vi "Drawing Proof Of Concept Early.vi"() -> ()   [LabVIEW 2021]
uses:
  <vilib>/Utility/inputDevices.llb/mouseAcquire.vi
  <vilib>/Utility/inputDevices.llb/closeMouse.vi
panel:
  in  "Clear Drawing":bool
  out "Robot Drawn So Far":cluster{i32[], i32[]}[](graph)
  in  "Cancel Drawing Queue":bool
  out "Obstacle Detected":bool
  out "Robot Vertical":dbl
  out "Robot Horizontal":dbl
  out "Chalk Force Readout":dbl
  out "Current Mouse Coordinates":T1
  out "Drawing":cluster{i32[], i32[]}[](graph)
  out "Mouse Status":cluster{"Clicked?":bool}
  in  "Emergency Stop":bool
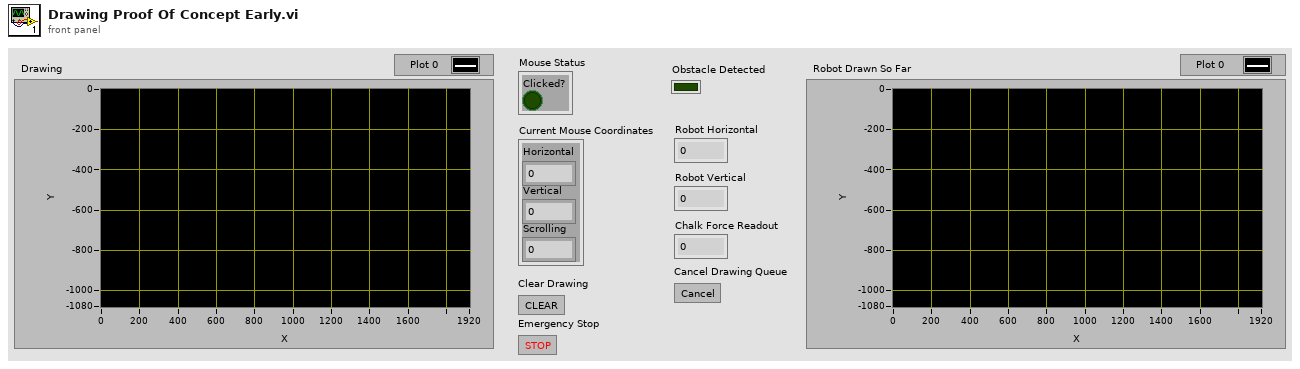
[diagram p1: front panel]
types:
  T1 = cluster{"Horizontal":i32, "Vertical":i32, "Scrolling":i32}
  T2 = cluster{"Horizontal Array":i32[], "Vertical Array":i32[]}
  T3 = cluster{"Horizontal Array":i32[], "Vertical Array":i32[]}[]
  T4 = cluster{"button 1":bool, "button 2":bool, "button 3":bool, "button 4":bool}
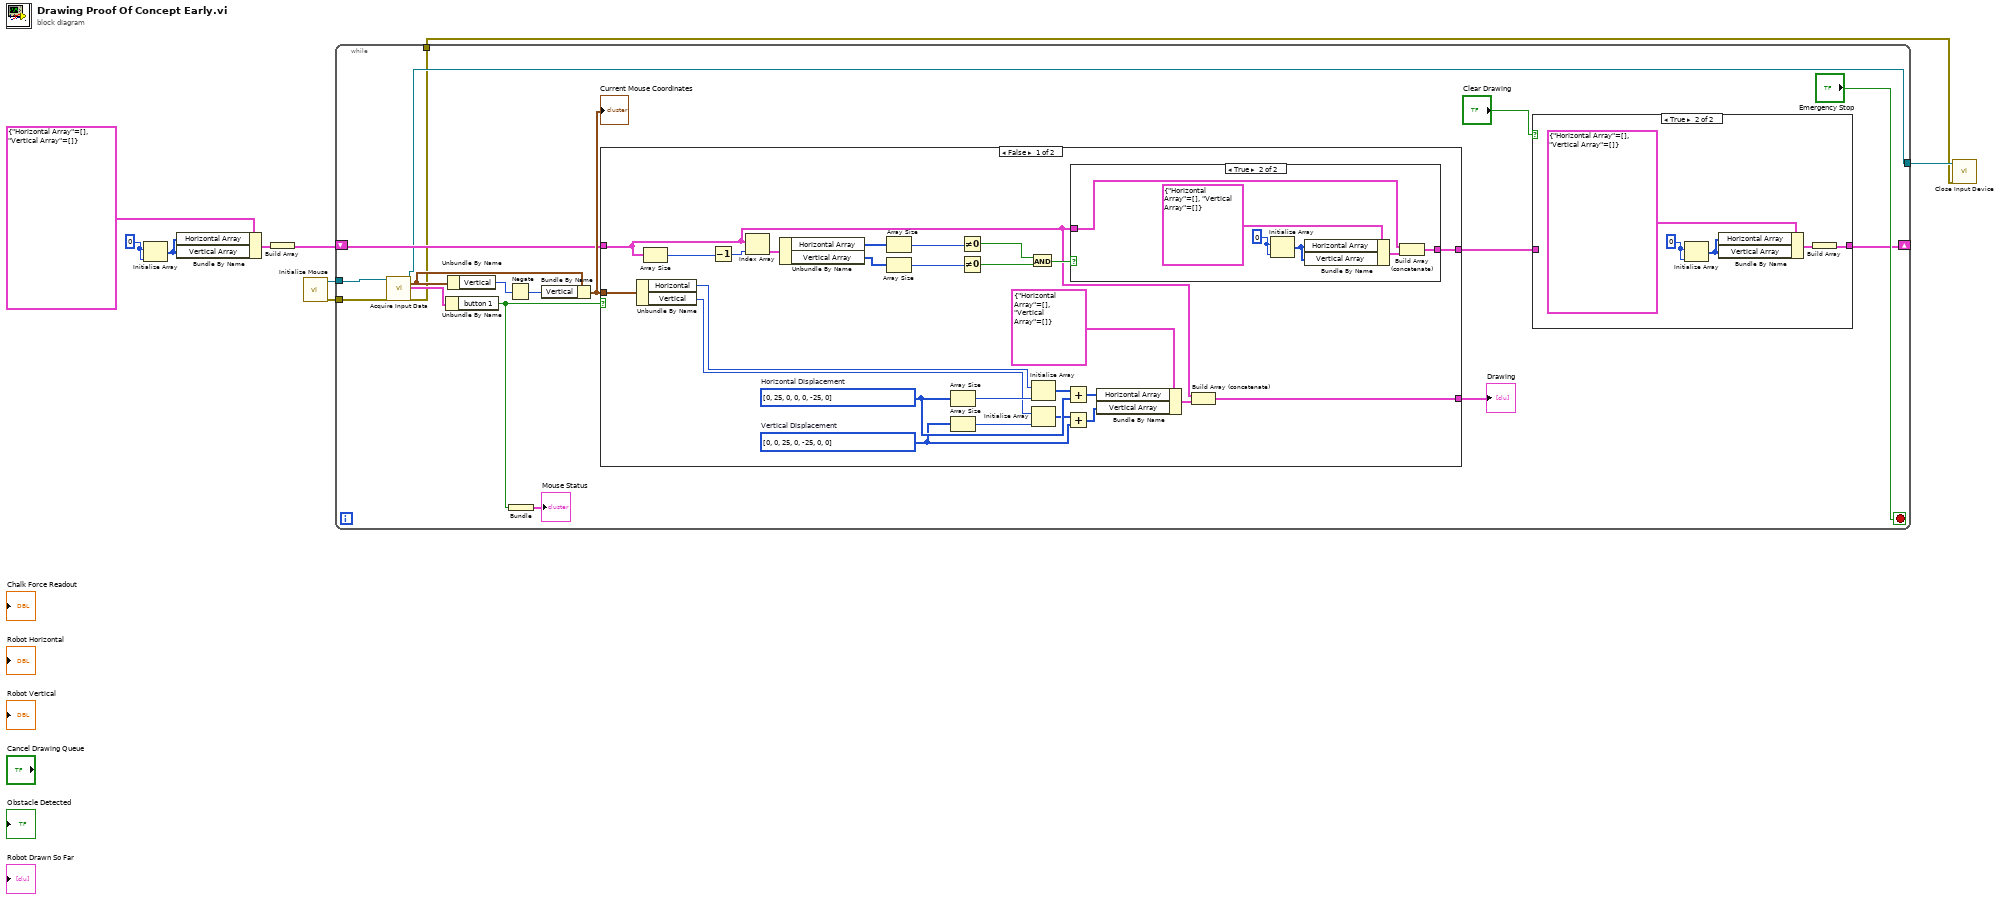
[diagram p0: block diagram]
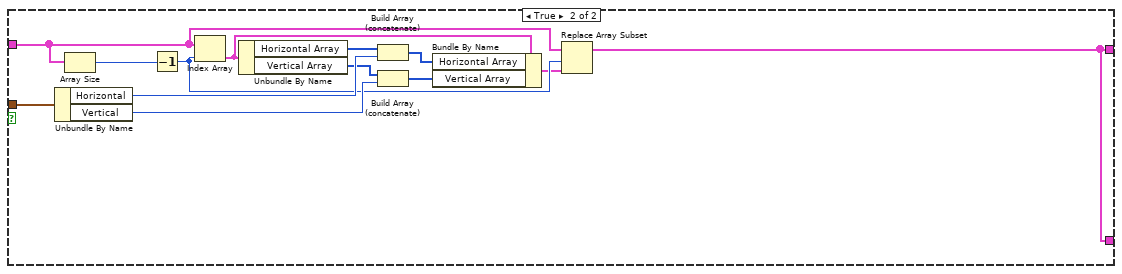
[diagram p4: hidden frame]
diagram:
  w5 = 0
  n1 = Initialize Array(w5, w5) -> (w3:i32[])
  n2 = Bundle By Name(cluster=T2 {"Horizontal Array"=[], "Vertical Array"=[]}, "Horizontal Array"=w3, "Vertical Array"=w3) -> (w6:T2)
  n3 = Build Array(w6) -> (w4:T3)
  n4 = call <vilib>:"Initialize Mouse.vi"() -> ("error out"=w8:errorcluster, "device ID"=w9:refnum<k1>)  [unwired: 10 in]
  n5 = while {
    tunnel: w9 -> [w25]
    tunnel: w8 -> [w24]
    shift-right: [w12] -> _
    shift-left: w4 -> [w16]
    tunnel: [w11] -> w2
    tunnel: [w10] -> w1
    stop <- "Emergency Stop" stop-if-true
    n6 = call-poly <vilib>:"Acquire Input Data.vi"("device ID"=w25, "error in (no error)"=w24) -> ("device ID"=w11:refnum<k1>, "axis info"=w22:T1, "button info"=w23:T4, "error out"=w10:errorcluster)  [unwired: 14 in]
    n7 = Unbundle By Name(w23) -> ("button 1"=w18:bool)
    n8 = Unbundle By Name(w22) -> ("Vertical"=w21:i32)
    n9 = Negate(x=w21) -> (-x=w20:i32)
    n10 = Bundle("button 1"=w18) -> (→"Mouse Status":cluster{"button 1":bool})  [unwired: 1 in]
    n11 = Bundle By Name(cluster=w22, "Vertical"=w20) -> (w17:T1)
    "Current Mouse Coordinates" <- w17
    n12 = case shown="False" w18 {
      tunnel: w16 -> [w45 w69]
      tunnel: w17 -> [w47 w78]
      tunnel: [w48 w66] -> w13
      tunnel: [w43 w66] -> w15
      frame False {
        w35 = i32[] [0, 0, 25, 0, -25, 0, 0]  # Vertical Displacement
        w37 = i32[] [0, 25, 0, 0, 0, -25, 0]  # Horizontal Displacement
        n13 = Unbundle By Name(w47) -> ("Horizontal"=w42:i32, "Vertical"=w40:i32)
        n14 = Array Size(array=w45) -> (size(s)=w56:i32)
        n15 = Decrement(x=w56) -> (x-1=w58:i32)
        n16 = Index Array(array=w45, index=w58) -> (element=w57:T2)
        n17 = Unbundle By Name(w57) -> ("Horizontal Array"=w55:i32[], "Vertical Array"=w54:i32[])
        n18 = Array Size(array=w55) -> (size(s)=w53:i32)
        n19 = Array Size(array=w54) -> (size(s)=w52:i32)
        n20 = Array Size(array=w37) -> (size(s)=w41:i32)
        n21 = Array Size(array=w35) -> (size(s)=w39:i32)
        n22 = Not Equal To 0?(x=w53) -> (x != 0?=w51:bool)
        n23 = Not Equal To 0?(x=w52) -> (x != 0?=w50:bool)
        n24 = And(x=w51, y=w50) -> (x .and. y?=w49:bool)
        n25 = Initialize Array(w42, w41) -> (w38:i32[])
        n26 = Initialize Array(w40, w39) -> (w36:i32[])
        n27 = Add(x=w38, y=w37) -> (x+y=w33:i32[])
        n28 = Add(x=w36, y=w35) -> (x+y=w34:i32[])
        n29 = case shown="True" w49 {
          tunnel: w45 -> [w59 w63]
          tunnel: [w59 w60] -> w48
          frame False {
          }
          frame True {
            w64 = 0
            n30 = Initialize Array(w64, w64) -> (w65:i32[])
            n31 = Bundle By Name(cluster=T2 {"Horizontal Array"=[], "Vertical Array"=[]}, "Horizontal Array"=w65, "Vertical Array"=w65) -> (w61:T2)
            n32 = Build Array (concatenate)(w63, w61) -> (w60:T3)
          }
        }
        n33 = Bundle By Name(cluster=T2 {"Horizontal Array"=[], "Vertical Array"=[]}, "Horizontal Array"=w33, "Vertical Array"=w34) -> (w44:T2)
        n34 = Build Array (concatenate)(w45, w44) -> (w43:T3)
      }
      frame True {
        n35 = Unbundle By Name(w78) -> ("Horizontal"=w75:i32, "Vertical"=w73:i32)
        n36 = Array Size(array=w69) -> (size(s)=w77:i32)
        n37 = Decrement(x=w77) -> (x-1=w68:i32)
        n38 = Index Array(array=w69, index=w68) -> (element=w72:T2)
        n39 = Unbundle By Name(w72) -> ("Horizontal Array"=w76:i32[], "Vertical Array"=w74:i32[])
        n40 = Build Array (concatenate)(w76, w75) -> (w71:i32[])
        n41 = Build Array (concatenate)(w74, w73) -> (w70:i32[])
        n42 = Bundle By Name(cluster=w72, "Horizontal Array"=w71, "Vertical Array"=w70) -> (w67:T2)
        n43 = Replace Array Subset(array=w69, new element=w67, index=w68) -> (w66:T3)
      }
    }
    "Drawing" <- w15
    n44 = case shown="True" "Clear Drawing" {
      tunnel: w13 -> [w27 _]
      tunnel: [w27 w28] -> w12
      frame False {
      }
      frame True {
        w30 = 0
        n45 = Initialize Array(w30, w30) -> (w32:i32[])
        n46 = Bundle By Name(cluster=T2 {"Horizontal Array"=[], "Vertical Array"=[]}, "Horizontal Array"=w32, "Vertical Array"=w32) -> (w31:T2)
        n47 = Build Array(w31) -> (w28:T3)
      }
    }
  }
  n48 = call-poly <vilib>:"Close Input Device.vi"("error in (no error)"=w1, "device ID"=w2) -> ()  [unwired: 8 in, 1 out]
